vi "SalvaImpostazioni_INPUT.vi"(10 "banco":i32=1) -> ()   [LabVIEW 2019]
uses:
  TypeDef/ClusterCaratteristicheMisura_INPUT.ctl
panel:
  in  "Stop":bool
  in  "Carica Impostazioni":bool
  out "Numero di misure":i32
  in  "Salva Impostazioni":bool
  in  "Array ClusterCaratteristicheMisura":T1[](array[typedef])
  # "RISERVATO AD \nUSO INTESYS"
  # "Dichiarare in questa sezione\ntutti gli ingressi analogici del sistema\n(sia fisici che virtuali come ad\nesempio dati acquisiti dal plc).\n\nPer ogni ingresso mettere a TRUE\nil tasto \"Scala?\" se si desidera riscalare\nil valore letto (inserire pertanto\nAi_min,Ai_max,Range,Offset)\n\nSe si seleziona il tasto \"SENSORE?\"\nil riscalamento non avverrà con i \ndati inseriti in questa sezione ma\ncon i dati di range ed offset del\nsensore associato all'ingresso\nnella apposita sezione del programma\n\nSe non vengono selezionati nè \n\"Scala?\" nè \"SENSORE\" il dato non\nverrà riscalato in alcun modo"
  # "ATTENZIONE :\nSE SI MODIFICA IL NOME DI UN\nINGRESSO ESISTENTE,\nBISOGNA POI RICREARE LA\nMAPPATURA \nINGRESSI-SENSORI-LINEE\nIN \"GESTIONE SENSORI.VI\""
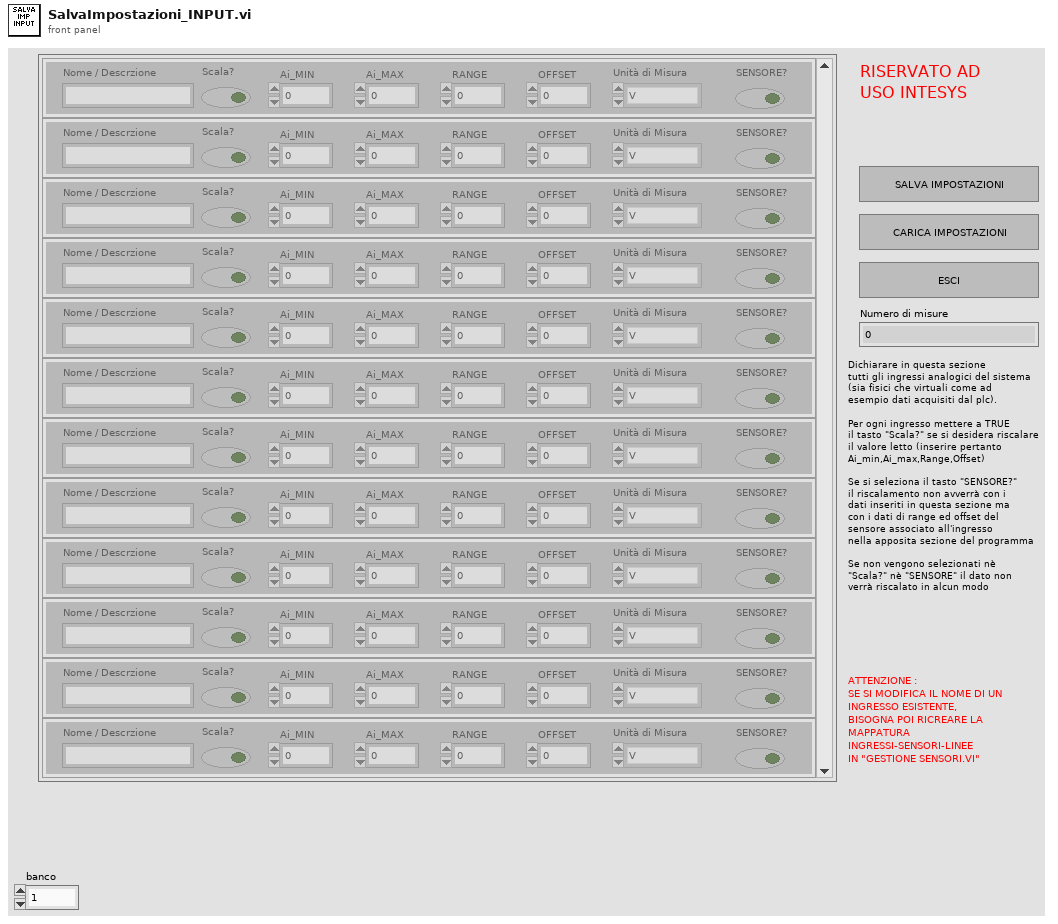
[diagram p1: front panel]
types:
  T1 = typedef "ClusterCaratteristicheMisura_INPUT.ctl" = cluster{"Nome / Descrzione":string, "Scala?":bool, "Ai_MIN":dbl, "Ai_MAX":dbl, "RANGE":dbl, "OFFSET":dbl, "Unità di Misura":T2, "SENSORE?":bool}
  T2 = typedef "UnitàMisura.ctl" = enum16{"V", "mA", "Bar", "RPM", "m3/s", "m3/min", "m3/h", "l/s", "l/min", "in3/min", "ft3/min", "gpm", "igpm", "igph", "%", "°C", "m", "Nm", "A"}
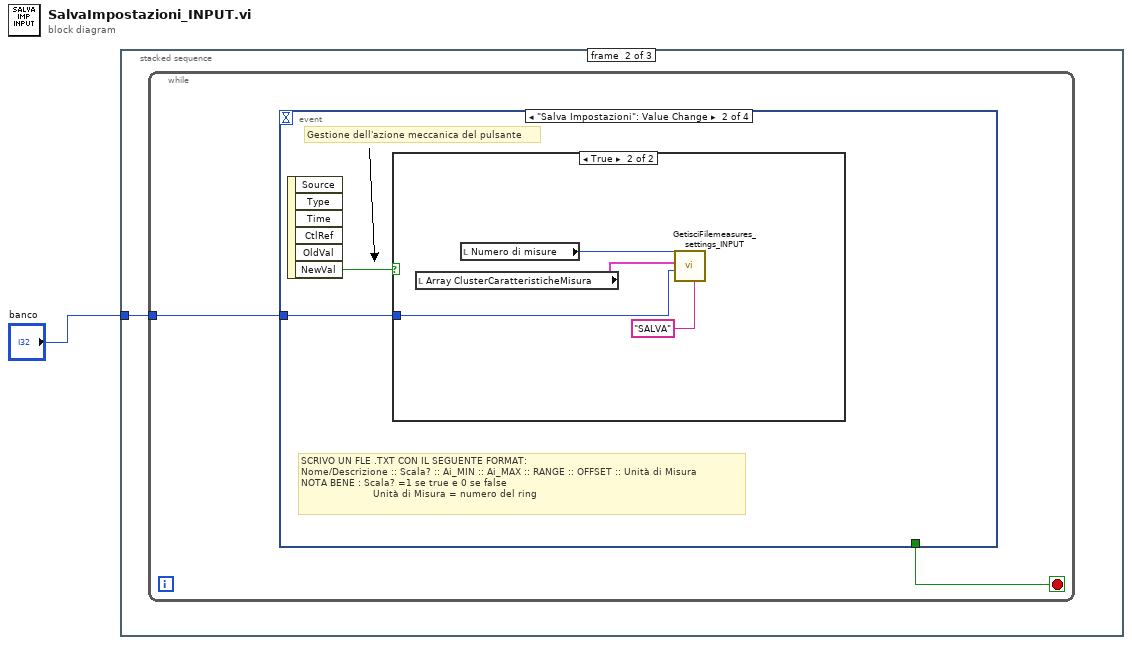
[diagram p0: block diagram]
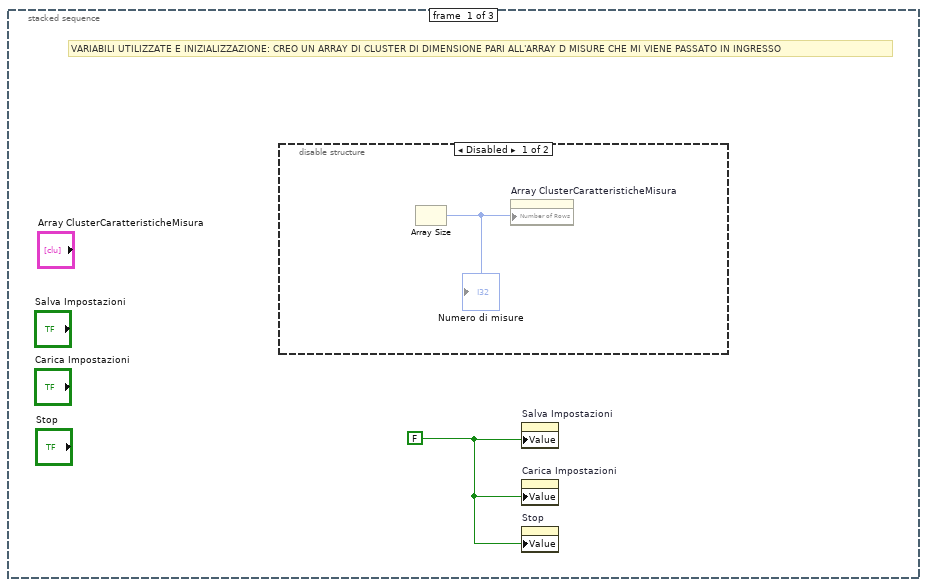
[diagram p2: hidden frame]
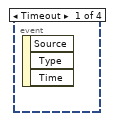
[diagram p4: hidden frame]
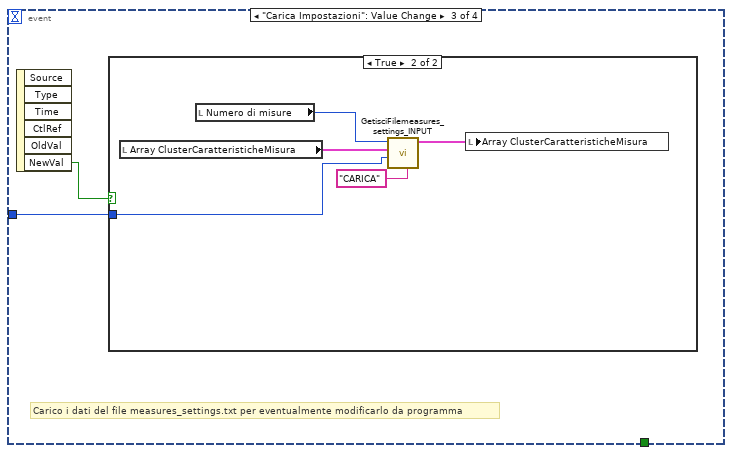
[diagram p6: hidden frame]
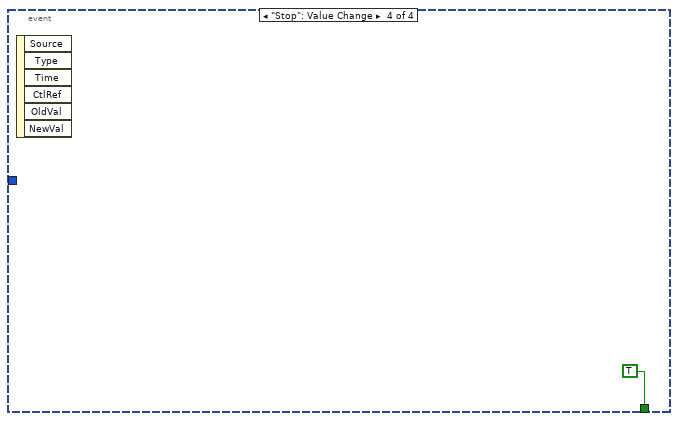
[diagram p8: hidden frame]
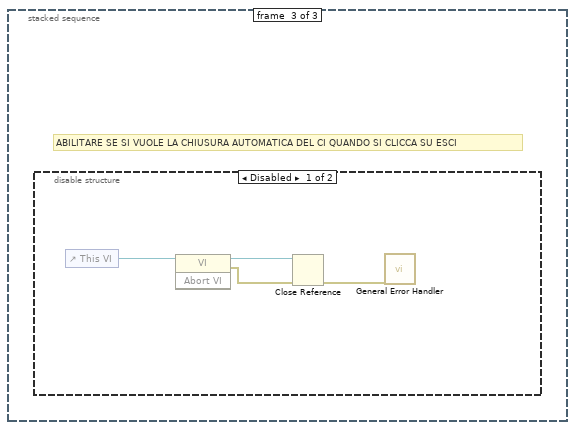
[diagram p9: hidden frame]
diagram:
  n1 = stacked-sequence {
    tunnel: "banco" -> [_ w5 _]
    frame #0 {
      w2 = FALSE ("Salva Impostazioni")
      # "VARIABILI UTILIZZATE E INIZIALIZZAZIONE: CREO UN ARRAY DI CLUSTER DI DIMENSIONE PARI ALL'ARRAY D MISURE CHE MI VIENE PASSATO IN INGRESSO"
      n2 = disable-structure shown="Disabled" {
        frame Disabled {
          n3 = Array Size() -> (array=w4:dbl[], size(s)=w3:i32)
          "Numero di misure" <- w3
          n4 = property on="Array ClusterCaratteristicheMisura" class="Arr (strict)"("Number of Rows"=w3) -> ()  [unwired: 2 in, 2 out]
        }
        frame Enabled {
        }
      }
      n5 = property on="Salva Impostazioni" class="Bool (strict)"("Value"=w2) -> ()  [unwired: 2 in, 2 out]
      n6 = property on="Carica Impostazioni" class="Bool (strict)"("Value"=w2) -> ()  [unwired: 2 in, 2 out]
      n7 = property on="Stop" class="Bool (strict)"("Value"=w2) -> ()  [unwired: 2 in, 2 out]
    }
    frame #1 {
      n8 = while {
        tunnel: w5 -> [w6]
        stop <- w7 stop-if-true
        n9 = event shown="[1] \"Salva Impostazioni\": Value Change" {
          selector: _ -> [_ _ _ _]
          dyn-events: _ -> [_ _ _ _]
          timeout: _ -> [_ _ _ _]
          tunnel: [_ _ _ TRUE] -> w7
          tunnel: w6 -> [_ w8 w14 _]
          event Timeout {
            n10 = event-data() -> ()  [unwired: 1 in, 3 out]
          }
          event "Salva Impostazioni": Value Change {
            # "Gestione dell'azione meccanica del pulsante"
            # "SCRIVO UN FLE .TXT CON IL SEGUENTE FORMAT:\nNome/Descrizione :: Scala? :: Ai_MIN :: Ai_MAX :: RANGE :: OFFSET :: Unità di Misura \nNOTA BENE : Scala? =1 se true e 0 se false\n                        Unità di Misura = numero del ring"
            n11 = event-data() -> ("NewVal"=w9:bool)  [unwired: 1 in, 5 out]
            n12 = case shown="True" w9 {
              tunnel: w8 -> [_ w10]
              frame False {
              }
              frame True {
                n13 = local read "Array ClusterCaratteristicheMisura"() -> (w12:T1[])
                n14 = local read "Numero di misure"() -> (w13:i32)
                n15 = call "GetisciFilemeasures_settings_INPUT.vi"("Numero Misure"=w13, "Array ClusterCaratteristicheMisura IN"=w12, "banco"=w10, "Azione"="SALVA") -> ()  [unwired: 6 in, 1 out]
              }
            }
          }
          event "Carica Impostazioni": Value Change {
            # "Carico i dati del file measures_settings.txt per eventualmente modificarlo da programma"
            n16 = event-data() -> ("NewVal"=w15:bool)  [unwired: 1 in, 5 out]
            n17 = case shown="True" w15 {
              tunnel: w14 -> [_ w16]
              frame False {
              }
              frame True {
                n18 = local read "Array ClusterCaratteristicheMisura"() -> (w19:T1[])
                n19 = local read "Numero di misure"() -> (w18:i32)
                n20 = call "GetisciFilemeasures_settings_INPUT.vi"("Numero Misure"=w18, "Array ClusterCaratteristicheMisura IN"=w19, "banco"=w16, "Azione"="CARICA") -> ("Array ClusterCaratteristicheMisura OUT"=w17:T1[])  [unwired: 6 in]
                n21 = local write "Array ClusterCaratteristicheMisura"(w17) -> ()
              }
            }
          }
          event "Stop": Value Change {
            n22 = event-data() -> ()  [unwired: 1 in, 6 out]
          }
        }
      }
    }
    frame #2 {
      # "ABILITARE SE SI VUOLE LA CHIUSURA AUTOMATICA DEL CI QUANDO SI CLICCA SU ESCI"
      n23 = disable-structure shown="Disabled" {
        frame Disabled {
          n24 = control-ref of="This VI"() -> (w25:refnum<vi>)
          n25 = invoke class="VI" method="Abort VI"(reference=w25) -> (reference out=w24:refnum<vi>, error out=w22:errorcluster)  [unwired: 2 in, 1 out]
          n26 = Close Reference(reference=w24, error in (no error)=w22) -> (error out=w23:errorcluster)
          n27 = call <vilib>:"General Error Handler.vi"("error in (no error)"=w23) -> ()  [unwired: 10 in, 5 out]
        }
        frame Enabled {
        }
      }
    }
  }
